vi "module.Layouts.vi"(4 "Min Value":i32=3 min=0 max=65535, 5 "camera.nit in":refnum<class "camera.lvclass">, 6 "Max Value":i32=97 min=1 max=65535, 7 "DVR":T4, 8 "error in":errorcluster, 10 "Image":T1(plugin-control), 11 "buffer":u16[][](array[numeric])) -> (0 "error out":errorcluster)   [LabVIEW 2020]
uses:
  _controls/element.ctl
  _controls/data.ctl
  camera/camera.lvclass
  _controls/data.ref.ctl
  <vilib>/vision/Image Controls.llb/IMAQ Image.ctl
  _controls/state.ctl
  _controls/data.vars.ctl
  _controls/save_options.ctl
  _controls/flip.ctl
  bus.ctl
  _controls/button.close.ctl
  <vilib>/Utility/file.llb/Read Delimited Spreadsheet (I64).vi
panel:
  in  "tab_button":bool
  in  "tab":enum32{"Image", "Array"}(tab)
  out "modules":T2[][](array[typedef])
  in  "position":T3(radio)
  in  "clear":bool
  in  "cancel":bool
  in  "save":bool
  in  "Columns":u8=1 min=1 max=10 step=1
  in  "Rows":u8=1 min=1 max=60 step=1
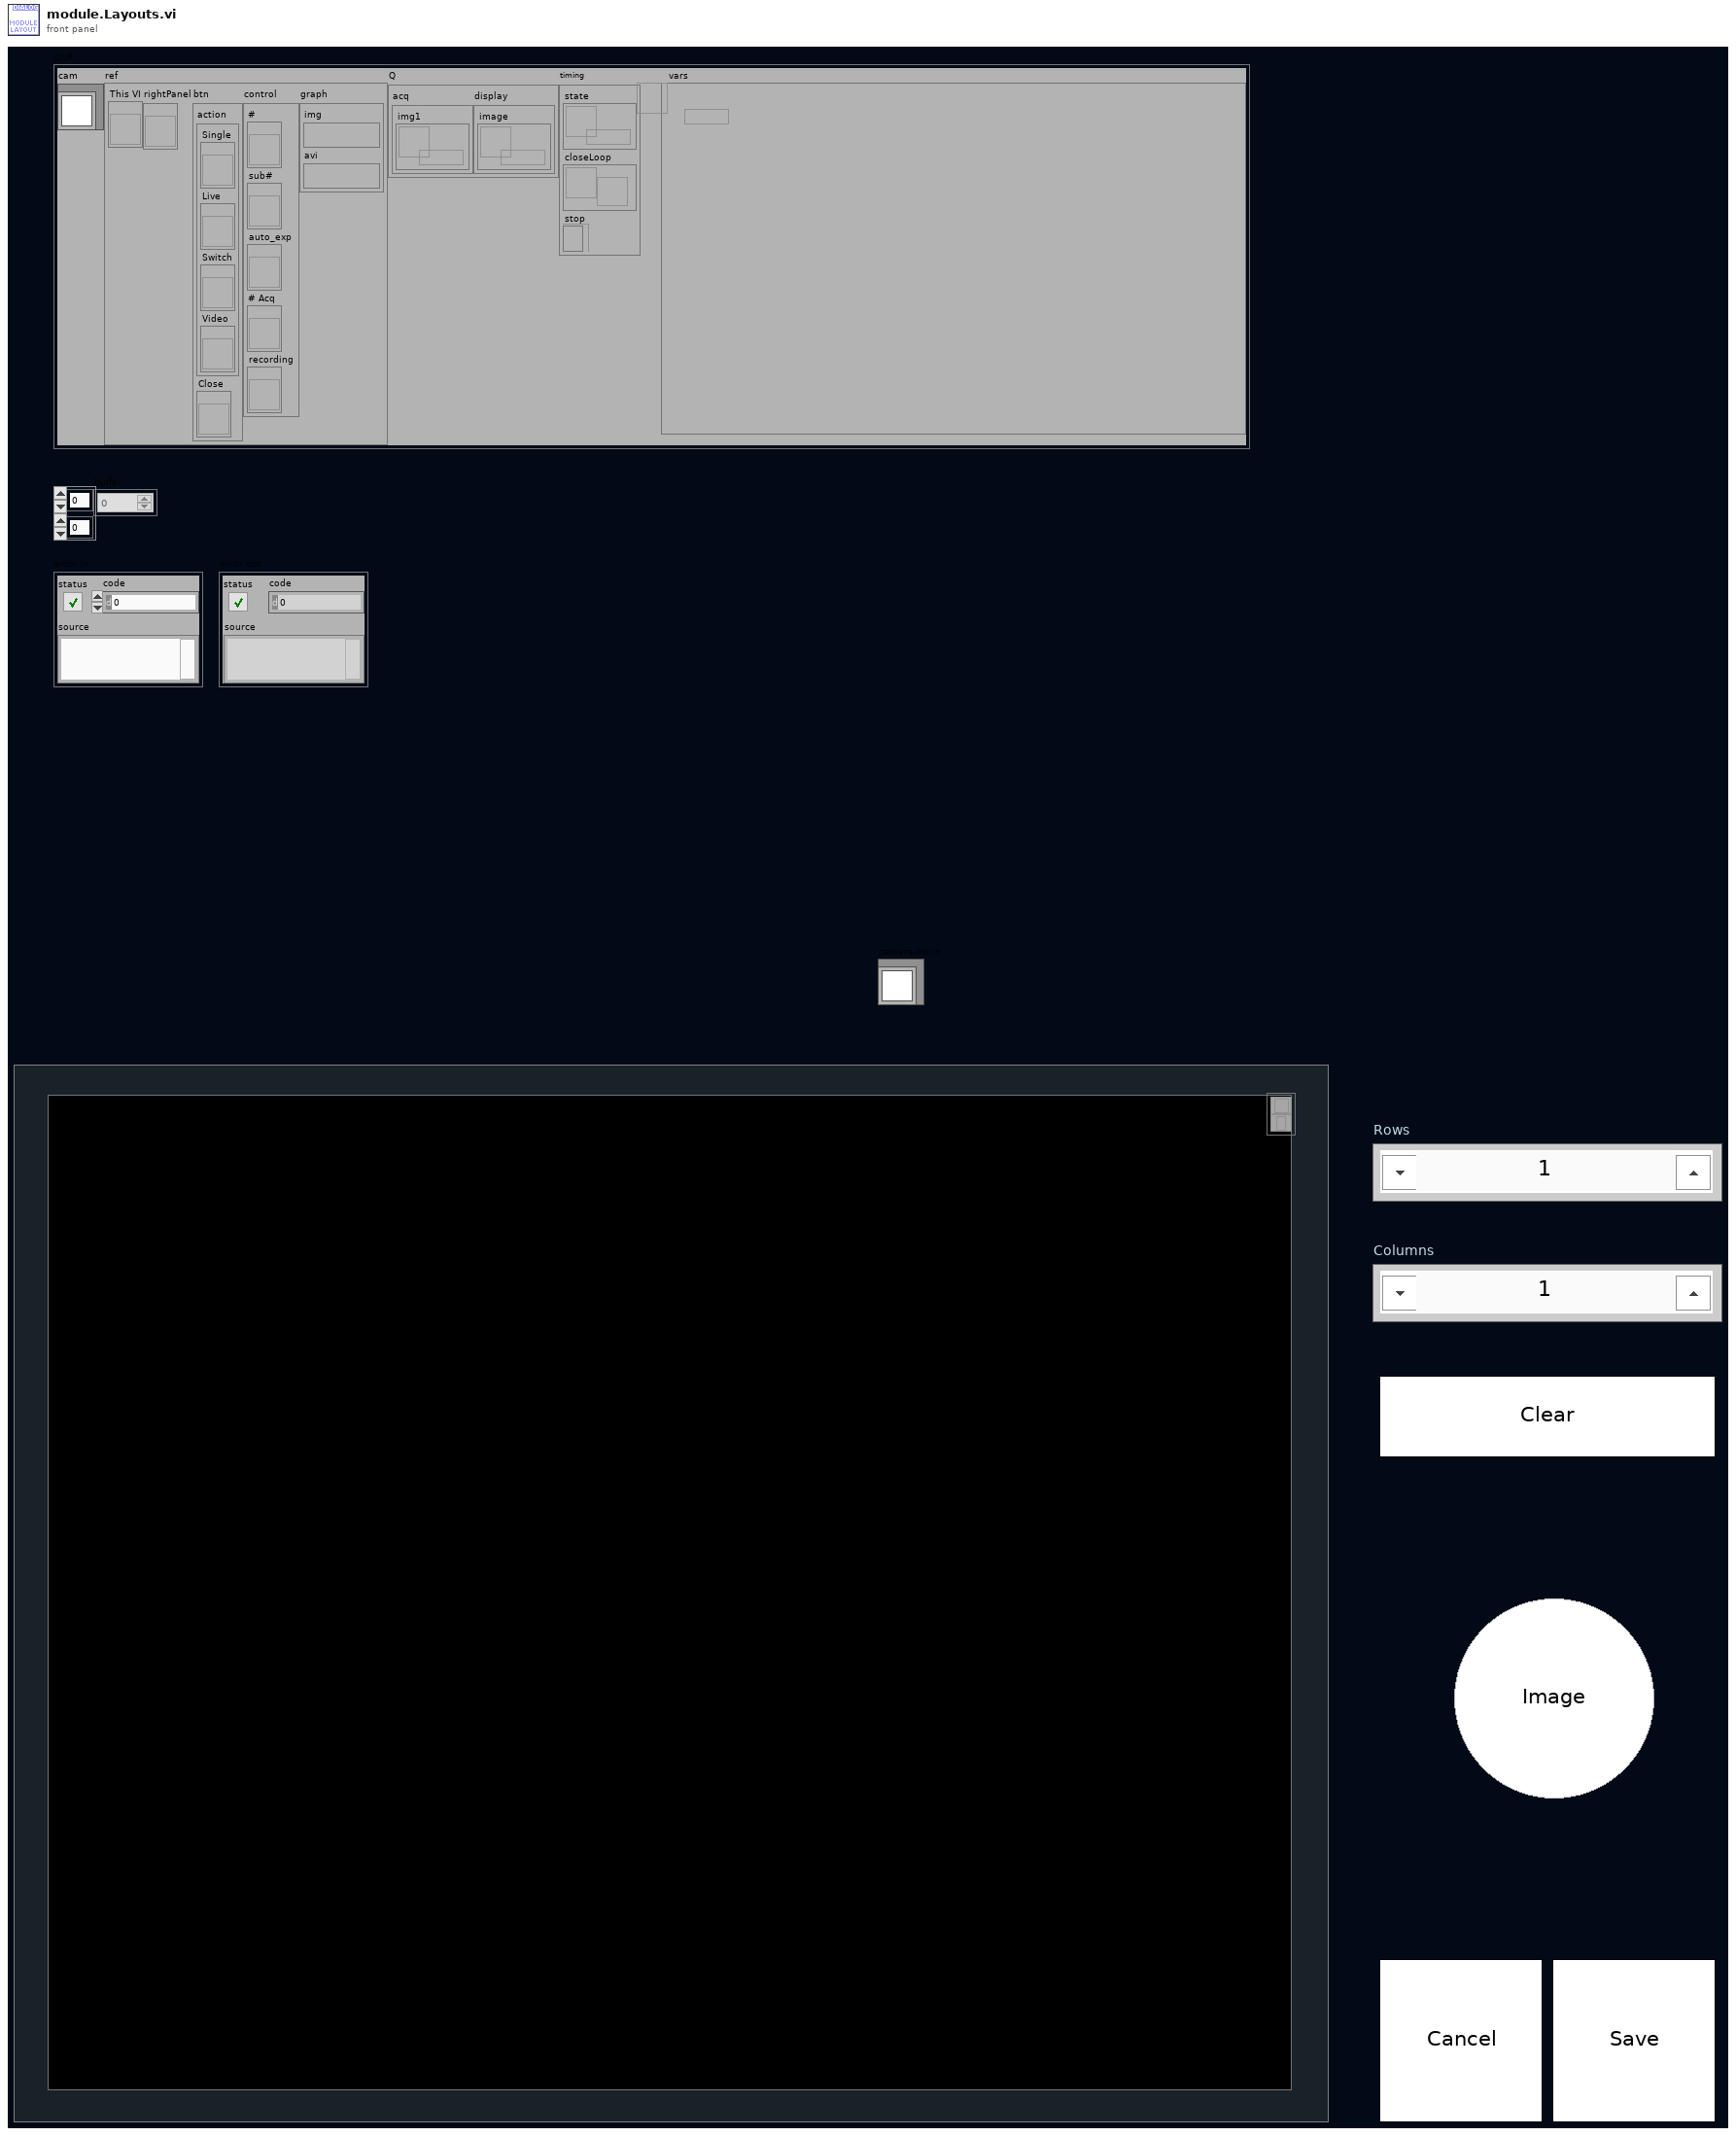
[diagram p1: front panel]
types:
  T1 = typedef "IMAQ Image.ctl" = refnum<image>
  T2 = typedef "element.ctl" = cluster{"Color Box":u32, "label":string}
  T3 = enum32{"1-10", "11-20", "21-30", "31-40", "41-50", "51-60"}
  T4 = typedef "data.ctl" = cluster{"cam":refnum<class "camera.lvclass">, "ref":T5, "Q":cluster{"acq":cluster{"img1":refnum<queue>}, "display":cluster{"image":refnum<queue>}}, "timing":cluster{"state":refnum<queue>, "closeLoop":refnum<notifier>, "stop":refnum<k4>}, "vars":refnum<data-value>}
  T5 = typedef "data.ref.ctl" = cluster{"This VI":refnum<vi>, "rightPanel":refnum<vi>, "btn":cluster{"action":cluster{"Single":refnum<vi>, "Live":refnum<vi>, "Switch":refnum<vi>, "Video":refnum<vi>}, "Close":refnum<vi>}, "control":cluster{"#":refnum<vi>, "sub#":refnum<vi>, "auto_exp":refnum<vi>, "# Acq":refnum<vi>, "recording":refnum<vi>}, "graph":cluster{"img":T1, "avi":T1}}
  T6 = typedef "bus.ctl" = cluster{"ref":cluster{"Columns":refnum<vi>, "rows":refnum<vi>, "position":refnum<vi>, "modules":refnum<vi>, "This VI":refnum<vi>}}
  T7 = typedef "button.close.ctl" = bool
  T8 = enum8{"Enabled", "Disabled", "Disabled and Grayed Out"}
  T9 = typedef "data.vars.ctl" = cluster{"save":cluster{"base_folder":cluster{"Folder":path, "tif":bool, "jpg":bool}, "module":string, "#":u32, "sub#":u8, "save.op":T10, "same?":bool, "Shift":enum16{"Single", "Leapfrog"}, "jpg?":bool, "flip":T11}, "acq":cluster{"# Acq":u16, "rotate":bool, "FPS":dbl, "Test Mode":bool}, "calib.manual":cluster{"BG":cluster{"Image":u16[][], "enabled?":bool}, "FF":cluster{"Image":u16[][], "enabled?":bool}}}
  T10 = typedef "save_options.ctl" = enum16{"Light", "Full"}
  T11 = typedef "flip.ctl" = cluster{"x":bool, "y":bool}
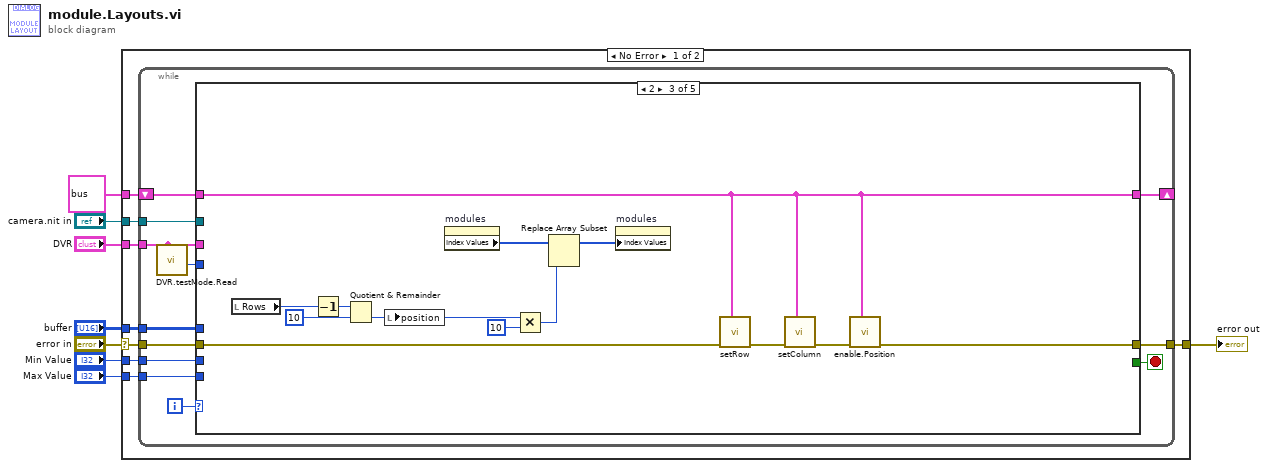
[diagram p0: block diagram]
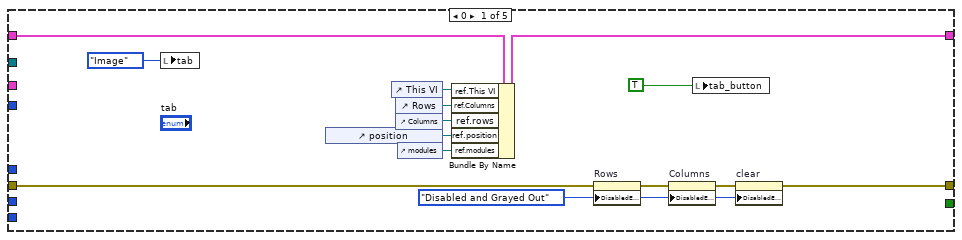
[diagram p2: hidden frame]
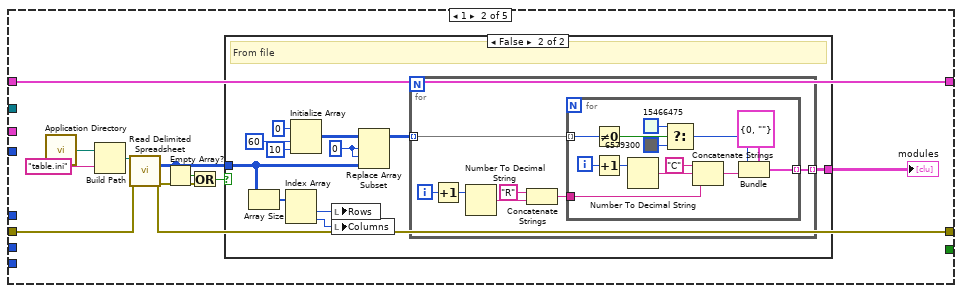
[diagram p3: hidden frame]
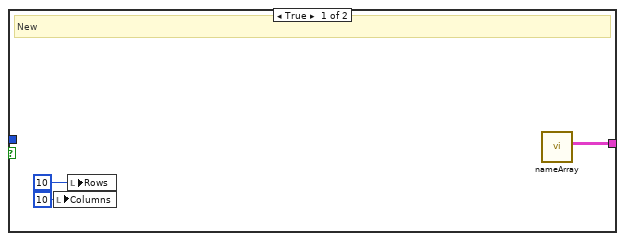
[diagram p4: hidden frame]
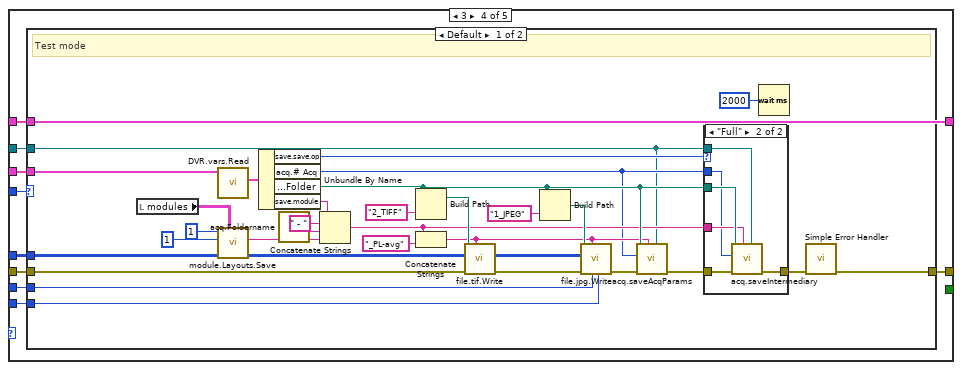
[diagram p5: hidden frame]
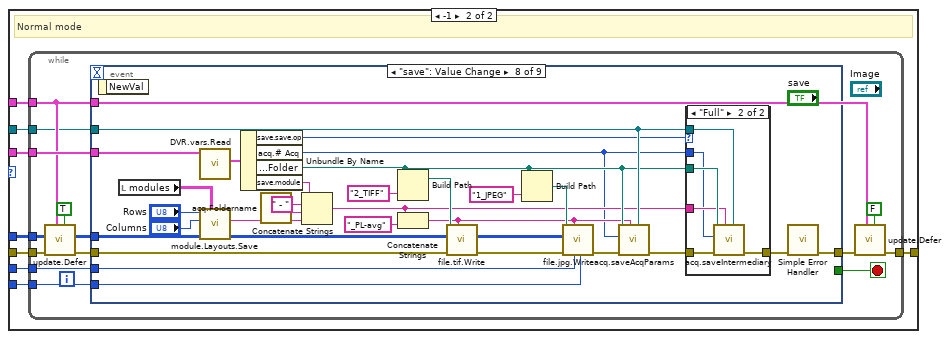
[diagram p7: hidden frame]
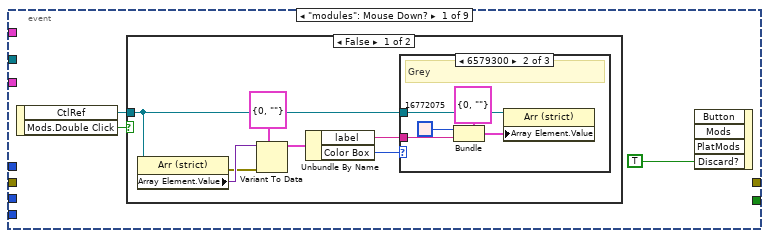
[diagram p8: hidden frame]
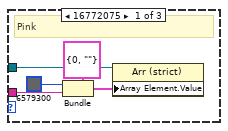
[diagram p9: hidden frame]
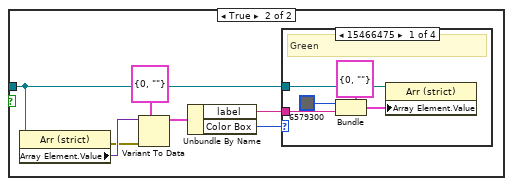
[diagram p11: hidden frame]
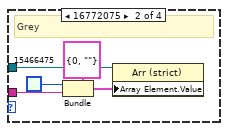
[diagram p12: hidden frame]
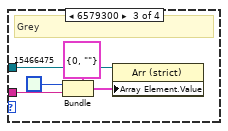
[diagram p13: hidden frame]
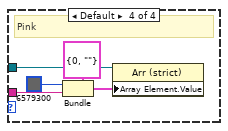
[diagram p14: hidden frame]
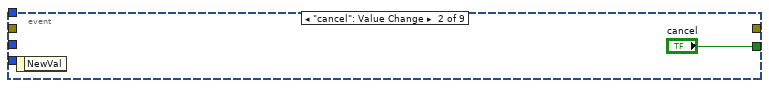
[diagram p15: hidden frame]
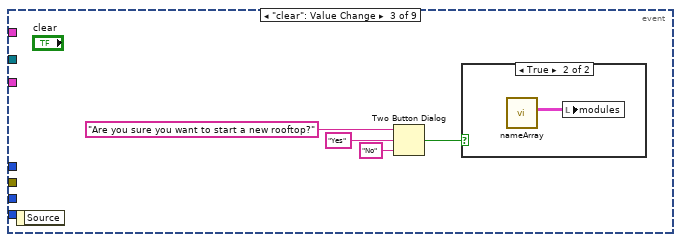
[diagram p16: hidden frame]
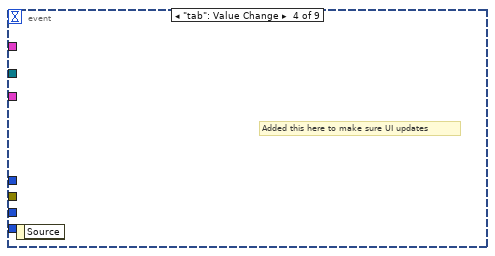
[diagram p18: hidden frame]
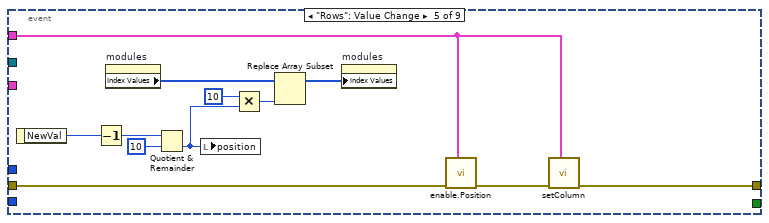
[diagram p19: hidden frame]
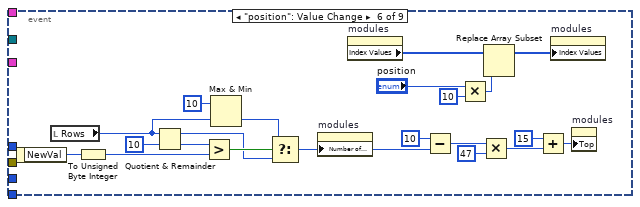
[diagram p20: hidden frame]
diagram:
  n1 = case shown="No Error" "error in" {
    selector: "error in" -> [w13 w308]
    tunnel: [w12 w308] -> w7
    tunnel: "buffer" -> [w16 _]
    tunnel: "DVR" -> [w15 _]
    tunnel: T6 {"ref"={"Columns"=refnum, "rows"=refnum, "position"=refnum, "modules"=refnum, "This VI"=refnum}} ("bus") -> [w14 _]
    tunnel: "camera.nit in" -> [w11 _]
    tunnel: "Max Value" -> [w10 _]
    tunnel: "Min Value" -> [w9 _]
    frame No Error {
      n2 = while {
        tunnel: w16 -> [w26]
        tunnel: w15 -> [w18]
        shift-right: [w24] -> _
        shift-left: w14 -> [w25]
        tunnel: w13 -> [w23]
        tunnel: [w22] -> w12
        tunnel: w11 -> [w21]
        tunnel: w10 -> [w20]
        tunnel: w9 -> [w19]
        i -> [w28]
        stop <- w27 stop-if-true
        n3 = call "DVR.testMode.Read.vi"("DVR in"=w18) -> ("timeout"=w17:i32)  [unwired: 10 in]
        n4 = case shown="2" w28 {
          tunnel: [_ _ _ _ TRUE] -> w27
          tunnel: w26 -> [_ _ _ w108 _]
          tunnel: w18 -> [_ _ _ w107 _]
          tunnel: w25 -> [w42 w45 w96 w104 w306]
          tunnel: [w41 w45 w96 w104 w306] -> w24
          tunnel: w23 -> [w32 w43 w99 w106 w305]
          tunnel: [w30 w44 w95 w105 w305] -> w22
          tunnel: w21 -> [_ _ _ w103 _]
          tunnel: w20 -> [_ _ _ w102 _]
          tunnel: w19 -> [_ _ _ w101 _]
          tunnel: w17 -> [_ _ _ w100 _]
          frame 0 {
            w29 = T8."Disabled and Grayed Out" ("Disabled")
            n5 = local write "tab"(enum32{"Image", "Array"}."Image" ("tab")) -> ()
            n6 = control-ref of="position"() -> (w40:refnum<vi>)
            n7 = control-ref of="This VI"() -> (w36:refnum<vi>)
            n8 = control-ref of="Rows"() -> (w39:refnum<vi>)
            n9 = control-ref of="Columns"() -> (w38:refnum<vi>)
            n10 = control-ref of="modules"() -> (w37:refnum<vi>)
            n11 = Bundle By Name(cluster=w42, "ref.This VI"=w36, "ref.Columns"=w39, "ref.rows"=w38, "ref.position"=w40, "ref.modules"=w37) -> (w41:T6)
            n12 = property on="Rows" class="DigNum (strict)"(error in=w32, "DisabledEnum"=w29) -> (error out=w33:errorcluster)  [unwired: 1 in, 1 out]
            n13 = property on="Columns" class="DigNum (strict)"(error in=w33, "DisabledEnum"=w29) -> (error out=w31:errorcluster)  [unwired: 1 in, 1 out]
            n14 = local write "tab_button"(TRUE ("cancel 2")) -> ()
            n15 = property on="clear" class="Bool"(error in=w31, "DisabledEnum"=w29) -> (error out=w30:errorcluster)  [unwired: 1 in, 1 out]
          }
          frame 1 {
            n16 = call <vilib>:"Application Directory.vi"() -> ("Application Directory"=w51:path)
            n17 = Build Path(base path=w51, name or relative path="table.ini" ("format (%d)")) -> (appended path=w49:path)
            n18 = call-poly <vilib>:"Read Delimited Spreadsheet.vi"("file path (dialog if empty)"=w49, "error in (no error)"=w43) -> ("all rows"=w47:i64[][], "error out"=w44:errorcluster)  [unwired: 8 in, 4 out]
            n19 = Empty Array?(array=w47) -> (empty?=w48:bool)
            n20 = Or(x=w48, y=w44) -> (x .or. y?=w46:bool)
            n21 = case shown="False" w46 {
              tunnel: [w53 w66] -> w52
              tunnel: w47 -> [_ w59]
              frame True {
                # "New"
                n22 = local write "Columns"(u8 10 ("Rows")) -> ()
                n23 = local write "Rows"(u8 10 ("Columns")) -> ()
                n24 = call "nameArray.vi"() -> ("Array"=w53:T2[][])  [unwired: 10 in, 1 out]
              }
              frame False {
                w64 = 0 ("index (row)")
                # "From file"
                n25 = Array Size(array=w59) -> (size(s)=w60:i32[])
                n26 = Index Array(array=w60) -> (element #1=w58:i32, element #2=w57:i32)  [unwired: 2 in]
                n27 = Initialize Array(u32 0 ("element"), 60 ("dimension size"), 10 ("dimension size")) -> (w61:u32[][])
                n28 = local write "Rows"(w58) -> ()
                n29 = local write "Columns"(w57) -> ()
                n30 = Replace Array Subset(array=w61, new element=w59, index (row)=w64, index (col)=w64) -> (w63:u32[][])
                n31 = for {
                  tunnel: [w71] -> w66 mode=indexing
                  tunnel: w63 -> [w69] mode=indexing
                  i -> [w73]
                  n32 = Increment(x=w73) -> (x+1=w70:i32)
                  n33 = Number To Decimal String(number=w70) -> (decimal integer string=w72:string)  [unwired: 1 in]
                  n34 = Concatenate Strings("R" ("string"), w72) -> (w68:string)
                  n35 = for {
                    tunnel: w68 -> [w83]
                    tunnel: [w84] -> w71 mode=indexing
                    tunnel: w69 -> [w82] mode=indexing
                    i -> [w76]
                    n36 = Not Equal To 0?(x=w82) -> (x != 0?=w81:bool)
                    n37 = Increment(x=w76) -> (x+1=w74:i32)
                    n38 = Number To Decimal String(number=w74) -> (decimal integer string=w75:string)  [unwired: 1 in]
                    n39 = Select(t=u32 15466475 ("Color Box"), s=w81, f=u32 6579300 ("Color Box")) -> (s? t:f=w79:u32)
                    n40 = Concatenate Strings("C" ("string"), w75, w83) -> (w86:string)
                    n41 = Bundle(cluster=T2 {"Color Box"=0, "label"=""} ("element"), "Color Box"=w79, "label"=w86) -> (w84:T2)
                  }
                }
              }
            }
            "modules" <- w52
          }
          frame 2 {
            n42 = local read "Rows"() -> (w93:u8)
            n43 = Decrement(x=w93) -> (x-1=w92:u8)
            n44 = Quotient & Remainder(x=w92, y=u8 10) -> (floor(x/y)=w88:u8)  [unwired: 1 out]
            n45 = local write "position"(w88) -> ()
            n46 = property on="modules" class="Arr (strict)"() -> ("Index Values"=w91:u32[])  [unwired: 2 in, 2 out]
            n47 = Multiply(x=w88, y=10) -> (x*y=w87:i32)
            n48 = Replace Array Subset(array=w91, new element=w87) -> (w90:u32[])  [unwired: 1 in]
            n49 = property on="modules" class="Arr (strict)"("Index Values"=w90) -> ()  [unwired: 2 in, 2 out]
            n50 = call "setRow.vi"("bus"=w96, "error in"=w99) -> ("error out"=w98:errorcluster)  [unwired: 9 in]
            n51 = call "setColumn.vi"("bus"=w96, "error in"=w98) -> ("error out"=w97:errorcluster)  [unwired: 9 in]
            n52 = call "enable.Position.vi"("bus"=w96, "error in"=w97) -> ("error out"=w95:errorcluster)  [unwired: 9 in]
          }
          frame 3 {
            n53 = case shown="Default" w100 {
              tunnel: w108 -> [w110 w153]
              tunnel: w107 -> [w111 w152]
              tunnel: w106 -> [w116 w151]
              tunnel: [w115 w150] -> w105
              tunnel: w104 -> [_ w149]
              tunnel: w103 -> [w112 w148]
              tunnel: w102 -> [w113 w147]
              tunnel: w101 -> [w114 w146]
              frame Default {
                # "Test mode"
                n54 = local read "modules"() -> (w130:T2[][])
                n55 = call "DVR.vars.Read.vi"("DVR.state"=w111) -> ("vars"=w134:T9)  [unwired: 9 in, 1 out]
                n56 = call "module.Layouts.Save.vi"("modules"=w130, "Columns"=u8 1 ("Columns 2"), "Rows"=u8 1 ("Rows 2")) -> ("spreadsheet string"=w129:string)  [unwired: 8 in]
                n57 = Unbundle By Name(w134) -> ("save.save.op"=w121:T10, "acq.# Acq"=w117:u16, "save.base_folder.Folder"=w122:path, "save.module"=w136:string)
                n58 = call "acq.Foldername.vi"() -> ("foldernme"=w133:string)  [unwired: 11 in]
                n59 = Concatenate Strings(w136, " - " ("string"), w133, w129) -> (w118:string)
                n60 = Build Path(base path=w122, name or relative path="2_TIFF" ("string")) -> (appended path=w132:path)
                n61 = Concatenate Strings(w118, "_PL-avg" ("string")) -> (w120:string)
                n62 = call "file.tif.Write.vi"("name"=w120, "error in"=w116, "u16 pixmap"=w110, "path"=w132) -> ("error out"=w126:errorcluster)  [unwired: 7 in]
                n63 = Build Path(base path=w122, name or relative path="1_JPEG" ("string")) -> (appended path=w127:path)
                n64 = call "file.jpg.Write.vi"("Max Value"=w113, "Min Value"=w114, "name"=w120, "error in"=w126, "u16 pixmap"=w110, "path"=w127) -> ("error out"=w125:errorcluster)  [unwired: 5 in]
                n65 = call "acq.saveAcqParams.vi"("camera in"=w112, "File name"=w120, "error in"=w125, "# Acq"=w117, "path"=w122) -> ("error out"=w124:errorcluster)  [unwired: 6 in]
                n66 = case shown="\"Full\"" w121 {
                  tunnel: w124 -> [w139 w145]
                  tunnel: [w139 w144] -> w123
                  tunnel: w112 -> [_ w143]
                  tunnel: w122 -> [_ w142]
                  tunnel: w118 -> [_ w141]
                  tunnel: w117 -> [_ w140]
                  frame "Light", Default {
                  }
                  frame "Full" {
                    n67 = call "acq.saveIntermediary.vi"("camera in"=w143, "name"=w141, "error in"=w145, "acq.# Acq"=w140, "path"=w142) -> ("error out"=w144:errorcluster)  [unwired: 6 in]
                  }
                }
                n68 = Wait (ms)(milliseconds to wait=u32 2000) -> ()  [unwired: 1 out]
                n69 = call <vilib>:"Simple Error Handler.vi"("error in (no error)"=w123) -> ("error out"=w115:errorcluster)  [unwired: 4 in, 4 out]
              }
              frame -1 {
                # "Normal mode"
                n70 = while {
                  tunnel: w153 -> [w165]
                  tunnel: w152 -> [w164]
                  tunnel: w151 -> [w161]
                  tunnel: [w162] -> w150
                  tunnel: w149 -> [w159]
                  tunnel: w148 -> [w156]
                  tunnel: w147 -> [w155]
                  tunnel: w146 -> [w154]
                  stop <- w166 stop-if-true
                  n71 = call "update.Defer.vi"("Defer Panel Updates"=TRUE, "bus in"=w159, "error in"=w161) -> ("error out"=w160:errorcluster)  [unwired: 8 in]
                  n72 = event shown="[7] \"save\": Value Change" {
                    selector: _ -> [_ _ _ _ _ _ _ _ _]
                    dyn-events: _ -> [_ _ _ _ _ _ _ _ _]
                    timeout: _ -> [_ _ _ _ _ _ _ _ _]
                    tunnel: [_ "cancel" _ _ _ _ _ T7 TRUE ("close") _] -> w166
                    tunnel: w165 -> [_ _ _ _ _ _ _ w274 _]
                    tunnel: w164 -> [_ _ _ _ _ _ _ w263 _]
                    tunnel: w160 -> [_ _ _ _ w225 _ w255 w271 w299]
                    tunnel: [_ _ _ _ w230 _ w254 w258 w294] -> w163
                    tunnel: w159 -> [_ _ _ _ w231 _ w253 _ _]
                    tunnel: w156 -> [_ _ _ _ _ _ _ w266 _]
                    tunnel: w155 -> [_ _ _ _ _ _ _ w256 _]
                    tunnel: w154 -> [_ _ _ _ _ _ _ w257 _]
                    event "modules": Mouse Down? {
                      n73 = event-data() -> ("CtlRef"=w169:refnum<vi>, "Mods.Double Click"=w168:bool)  [unwired: 1 in]
                      n74 = case shown="False" w168 {
                        tunnel: w169 -> [w171 w188]
                        frame False {
                          n75 = property class="Arr (strict)"(reference=w171) -> (error out=w172:errorcluster, "Array Element.Value"=w176:variant)  [unwired: 1 in, 1 out]
                          n76 = Variant To Data(error in=w172, type=T2 {"Color Box"=0, "label"=""} ("element"), Variant=w176) -> (data=w175:T2)  [unwired: 1 out]
                          n77 = Unbundle By Name(w175) -> ("label"=w174:string, "Color Box"=w170:u32)
                          n78 = case shown="6579300" w170 {
                            tunnel: w171 -> [w181 w186 _]
                            tunnel: w174 -> [w178 w183 _]
                            frame 16772075 {
                              # "Pink"
                              n79 = Bundle(cluster=T2 {"Color Box"=0, "label"=""} ("element"), "Color Box"=u32 6579300, "label"=w178) -> (w177:T2)
                              n80 = property class="Arr (strict)"(reference=w181, "Array Element.Value"=w177) -> ()  [unwired: 1 in, 2 out]
                            }
                            frame 6579300 {
                              # "Grey"
                              n81 = Bundle(cluster=T2 {"Color Box"=0, "label"=""} ("element"), "Color Box"=u32 16772075, "label"=w183) -> (w182:T2)
                              n82 = property class="Arr (strict)"(reference=w186, "Array Element.Value"=w182) -> ()  [unwired: 1 in, 2 out]
                            }
                            frame Default {
                              # "Default"
                            }
                          }
                        }
                        frame True {
                          n83 = property class="Arr (strict)"(reference=w188) -> (error out=w189:errorcluster, "Array Element.Value"=w193:variant)  [unwired: 1 in, 1 out]
                          n84 = Variant To Data(error in=w189, type=T2 {"Color Box"=0, "label"=""} ("element"), Variant=w193) -> (data=w192:T2)  [unwired: 1 out]
                          n85 = Unbundle By Name(w192) -> ("label"=w191:string, "Color Box"=w187:u32)
                          n86 = case shown="15466475" w187 {
                            tunnel: w188 -> [w198 w203 w208 w213]
                            tunnel: w191 -> [w196 w201 w205 w210]
                            frame 15466475 {
                              # "Green"
                              n87 = Bundle(cluster=T2 {"Color Box"=0, "label"=""} ("element"), "Color Box"=u32 6579300, "label"=w196) -> (w195:T2)
                              n88 = property class="Arr (strict)"(reference=w198, "Array Element.Value"=w195) -> ()  [unwired: 1 in, 2 out]
                            }
                            frame 16772075 {
                              # "Grey"
                              n89 = Bundle(cluster=T2 {"Color Box"=0, "label"=""} ("element"), "Color Box"=u32 15466475, "label"=w201) -> (w200:T2)
                              n90 = property class="Arr (strict)"(reference=w203, "Array Element.Value"=w200) -> ()  [unwired: 1 in, 2 out]
                            }
                            frame 6579300 {
                              # "Grey"
                              n91 = Bundle(cluster=T2 {"Color Box"=0, "label"=""} ("element"), "Color Box"=u32 15466475, "label"=w205) -> (w204:T2)
                              n92 = property class="Arr (strict)"(reference=w208, "Array Element.Value"=w204) -> ()  [unwired: 1 in, 2 out]
                            }
                            frame Default {
                              # "Pink"
                              n93 = Bundle(cluster=T2 {"Color Box"=0, "label"=""} ("element"), "Color Box"=u32 6579300, "label"=w210) -> (w209:T2)
                              n94 = property class="Arr (strict)"(reference=w213, "Array Element.Value"=w209) -> ()  [unwired: 1 in, 2 out]
                            }
                          }
                        }
                      }
                      n95 = event-data("Discard?"=TRUE) -> ()  [unwired: 4 in, 1 out]
                    }
                    event "cancel": Value Change {
                      n96 = event-data() -> ()  [unwired: 1 in, 1 out]
                    }
                    event "clear": Value Change {
                      n97 = event-data() -> ()  [unwired: 1 in, 1 out]
                      n98 = Two Button Dialog(message="Are you sure you want to start a new rooftop?", 1:"No" ("F button name (\"Cancel\")"), 2:"Yes" ("T button name (\"OK\")")) -> (T button?=w215:bool)
                      n99 = case shown="True" w215 {
                        frame False {
                        }
                        frame True {
                          n100 = call "nameArray.vi"() -> ("Array"=w219:T2[][])  [unwired: 10 in, 1 out]
                          n101 = local write "modules"(w219) -> ()
                        }
                      }
                    }
                    event "tab": Value Change {
                      # "Added this here to make sure UI updates"
                      n102 = event-data() -> ()  [unwired: 1 in, 1 out]
                    }
                    event "Rows": Value Change {
                      n103 = event-data() -> ("NewVal"=w228:u8)  [unwired: 1 in]
                      n104 = Decrement(x=w228) -> (x-1=w227:u8)
                      n105 = property on="modules" class="Arr (strict)"() -> ("Index Values"=w224:u32[])  [unwired: 2 in, 2 out]
                      n106 = Quotient & Remainder(x=w227, y=u8 10) -> (floor(x/y)=w222:u8)  [unwired: 1 out]
                      n107 = local write "position"(w222) -> ()
                      n108 = Multiply(x=u8 10 ("y"), y=w222) -> (x*y=w221:u8)
                      n109 = Replace Array Subset(array=w224, new element=w221) -> (w223:u32[])  [unwired: 1 in]
                      n110 = property on="modules" class="Arr (strict)"("Index Values"=w223) -> ()  [unwired: 2 in, 2 out]
                      n111 = call "enable.Position.vi"("bus"=w231, "error in"=w225) -> ("error out"=w229:errorcluster)  [unwired: 9 in]
                      n112 = call "setColumn.vi"("bus"=w231, "error in"=w229) -> ("error out"=w230:errorcluster)  [unwired: 9 in]
                    }
                    event "position": Value Change {
                      n113 = event-data() -> ("NewVal"=w247:T3)  [unwired: 1 in]
                      n114 = local read "Rows"() -> (w242:u8)
                      n115 = To Unsigned Byte Integer(number=w247) -> (unsigned 8bit integer=w245:u8)
                      n116 = Quotient & Remainder(x=w242, y=u8 10 ("x")) -> (x-y*floor(x/y)=w240:u8, floor(x/y)=w244:u8)
                      n117 = Greater?(x=w244, y=w245) -> (0:w243:bool)
                      n118 = Max & Min(x=u8 10, y=w242) -> (min(x,y)=w239:u8)  [unwired: 1 out]
                      n119 = Select(t=w239, s=w243, f=w240) -> (s? t:f=w233:u8)
                      n120 = property on="modules" class="Arr (strict)"("Number of Rows"=w233) -> ()  [unwired: 2 in, 2 out]
                      n121 = property on="modules" class="Arr (strict)"() -> ("Index Values"=w252:u32[])  [unwired: 2 in, 2 out]
                      n122 = Subtract(x=10, y=w233) -> (x-y=w238:i32)
                      n123 = Multiply(x="position", y=10) -> (x*y=w250:u32)
                      n124 = Multiply(x=w238, y=47) -> (x*y=w236:i32)
                      n125 = Replace Array Subset(array=w252, new element=w250) -> (w251:u32[])  [unwired: 1 in]
                      n126 = Add(x=15, y=w236) -> (x+y=w232:i32)
                      n127 = property on="modules" class="Arr (strict)"("Index Values"=w251) -> ()  [unwired: 2 in, 2 out]
                      n128 = property on="modules" class="Arr (strict)"("Top"=w232) -> ()  [unwired: 2 in, 2 out]
                    }
                    event "Columns": Value Change {
                      n129 = event-data() -> ()  [unwired: 1 in, 1 out]
                      n130 = call "setRow.vi"("bus"=w253, "error in"=w255) -> ("error out"=w254:errorcluster)  [unwired: 9 in]
                    }
                    event "save": Value Change {
                      n131 = event-data() -> ()  [unwired: 1 in, 1 out]
                      n132 = local read "modules"() -> (w276:T2[][])
                      n133 = call "DVR.vars.Read.vi"("DVR.state"=w263) -> ("vars"=w280:T9)  [unwired: 9 in, 1 out]
                      n134 = call "module.Layouts.Save.vi"("modules"=w276, "Columns"="Columns", "Rows"="Rows") -> ("spreadsheet string"=w275:string)  [unwired: 8 in]
                      n135 = Unbundle By Name(w280) -> ("save.save.op"=w264:T10, "acq.# Acq"=w259:u16, "save.base_folder.Folder"=w265:path, "save.module"=w282:string)
                      n136 = call "acq.Foldername.vi"() -> ("foldernme"=w279:string)  [unwired: 11 in]
                      n137 = Concatenate Strings(w282, " - " ("string"), w279, w275) -> (w260:string)
                      n138 = Build Path(base path=w265, name or relative path="2_TIFF" ("string")) -> (appended path=w278:path)
                      n139 = Concatenate Strings(w260, "_PL-avg" ("string")) -> (w262:string)
                      n140 = call "file.tif.Write.vi"("name"=w262, "error in"=w271, "u16 pixmap"=w274, "path"=w278) -> ("error out"=w270:errorcluster)  [unwired: 7 in]
                      n141 = Build Path(base path=w265, name or relative path="1_JPEG" ("string")) -> (appended path=w272:path)
                      n142 = call "file.jpg.Write.vi"("Max Value"=w256, "Min Value"=w257, "name"=w262, "error in"=w270, "u16 pixmap"=w274, "path"=w272) -> ("error out"=w269:errorcluster)  [unwired: 5 in]
                      n143 = call "acq.saveAcqParams.vi"("camera in"=w266, "File name"=w262, "error in"=w269, "# Acq"=w259, "path"=w265) -> ("error out"=w268:errorcluster)  [unwired: 6 in]
                      n144 = case shown="\"Full\"" w264 {
                        tunnel: w268 -> [w286 w292]
                        tunnel: [w286 w291] -> w267
                        tunnel: w266 -> [_ w290]
                        tunnel: w265 -> [_ w289]
                        tunnel: w260 -> [_ w288]
                        tunnel: w259 -> [_ w287]
                        frame "Light", Default {
                        }
                        frame "Full" {
                          n145 = call "acq.saveIntermediary.vi"("camera in"=w290, "name"=w288, "error in"=w292, "acq.# Acq"=w287, "path"=w289) -> ("error out"=w291:errorcluster)  [unwired: 6 in]
                        }
                      }
                      n146 = call <vilib>:"Simple Error Handler.vi"("error in (no error)"=w267) -> ("error out"=w258:errorcluster)  [unwired: 4 in, 4 out]
                    }
                    event "tab_button": Value Change {
                      n147 = event-data() -> ()  [unwired: 1 in, 1 out]
                      n148 = Select(t=enum32{"Image", "Array"}."Image" ("tab"), s="tab_button", f=enum32{"Image", "Array"}."Array") -> (s? t:f=w302:enum32{"Image", "Array"})
                      n149 = Select(t=T8."Disabled and Grayed Out" ("Disabled"), s="tab_button", f=T8."Enabled") -> (s? t:f=w293:T8)
                      n150 = property on="Rows" class="DigNum (strict)"(error in=w299, "DisabledEnum"=w293) -> (error out=w300:errorcluster)  [unwired: 1 in, 1 out]
                      n151 = local write "tab"(w302) -> ()
                      n152 = property on="Columns" class="DigNum (strict)"(error in=w300, "DisabledEnum"=w293) -> (error out=w295:errorcluster)  [unwired: 1 in, 1 out]
                      n153 = property on="clear" class="Bool"(error in=w295, "DisabledEnum"=w293) -> (error out=w294:errorcluster)  [unwired: 1 in, 1 out]
                    }
                  }
                  n154 = call "update.Defer.vi"("Defer Panel Updates"=FALSE, "bus in"=w159, "error in"=w163) -> ("error out"=w162:errorcluster)  [unwired: 8 in]
                }
              }
            }
          }
          frame Default {
            n155 = local write "tab"(enum32{"Image", "Array"}."Image" ("tab")) -> ()
          }
        }
      }
    }
    frame Error {
    }
  }
  "error out" <- w7
